vi "Example Callback - TouchState Callback.vi"(4 "TouchState":refnum<user-event>, 5 "Event Data":cluster{"sender":refnum<k24>, "state":i32}, 6 "Control Ref":refnum<k24>, 7 "Event Common Data":T1) -> ()   [LabVIEW 2010]
uses:
  C:/tf/play/labview/Tinkerforge.dll
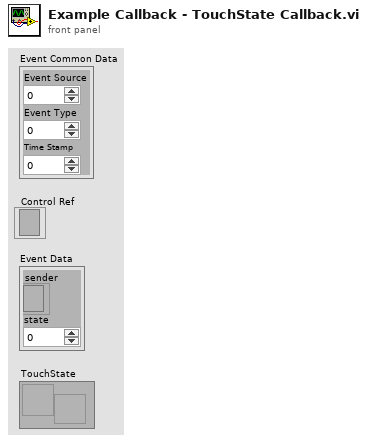
[diagram p1: front panel]
types:
  T1 = cluster{"Event Source":i32, "Event Type":u32, "Time Stamp":u32}
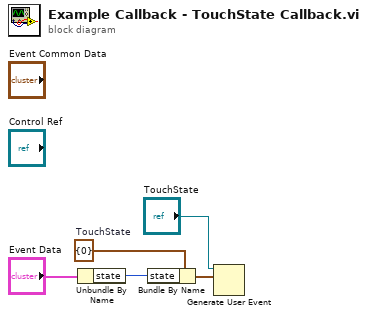
[diagram p0: block diagram]
diagram:
  w3 = cluster{"state":i32} {"state"=0}  # TouchState
  n1 = Unbundle By Name("Event Data") -> ("state"=w2:i32)
  n2 = Bundle By Name(cluster=w3, "state"=w2) -> (w5:cluster{"state":i32})
  n3 = Generate User Event(user event="TouchState", event data cluster=w5) -> ()  [unwired: 1 in, 2 out]
